vi "Resistomat_2316_2.vi"(0 "Scala resistomat":u16(ring)=5 items=["2 mOhm", "20 mOhm", "200 mOhm", "2 Ohm", "20 Ohm", "200 Ohm", "2 KOhm", "20 KOhm", "200 KOhm"], 1 "instrument ID":i32, 2 "N meas stab":i32=10, 3 "Precisione":dbl=0.005 format="%#_13g", 4 "T after start":u32=11, 5 "Time bef err":dbl=3.0, 7 "error out":errorcluster, 8 "COM-Port (0)":i32=3 min=1 max=32 step=1, 12 "Sing?":bool) -> (20 "seconds since 1Jan1904":timestamp, 21 "Measuring Value (ohm)":dbl, 25 "errore resistomat":bool, 27 "error out 2":errorcluster)   [LabVIEW 2019]
uses:
  Stop lettura res.vi
panel:
  in  "milliseconds to wait":u32=100
  out "Instrument Answers":string
  in  "Numeric 2":i32=5
  out "Numeric":i32
  in  "ms to wait":u32=100
  out "Measuring Value":dbl
  in  "array misure":dbl[](array[numeric])
  out "Scala resistomat 2":u16
  out "t":i32
  out "x .and. y?":bool
  out "x-y":dbl
  out "questionable status register":bool[](array[boolean])
  out "oper status register":bool[](array[boolean])
  out "error":bool
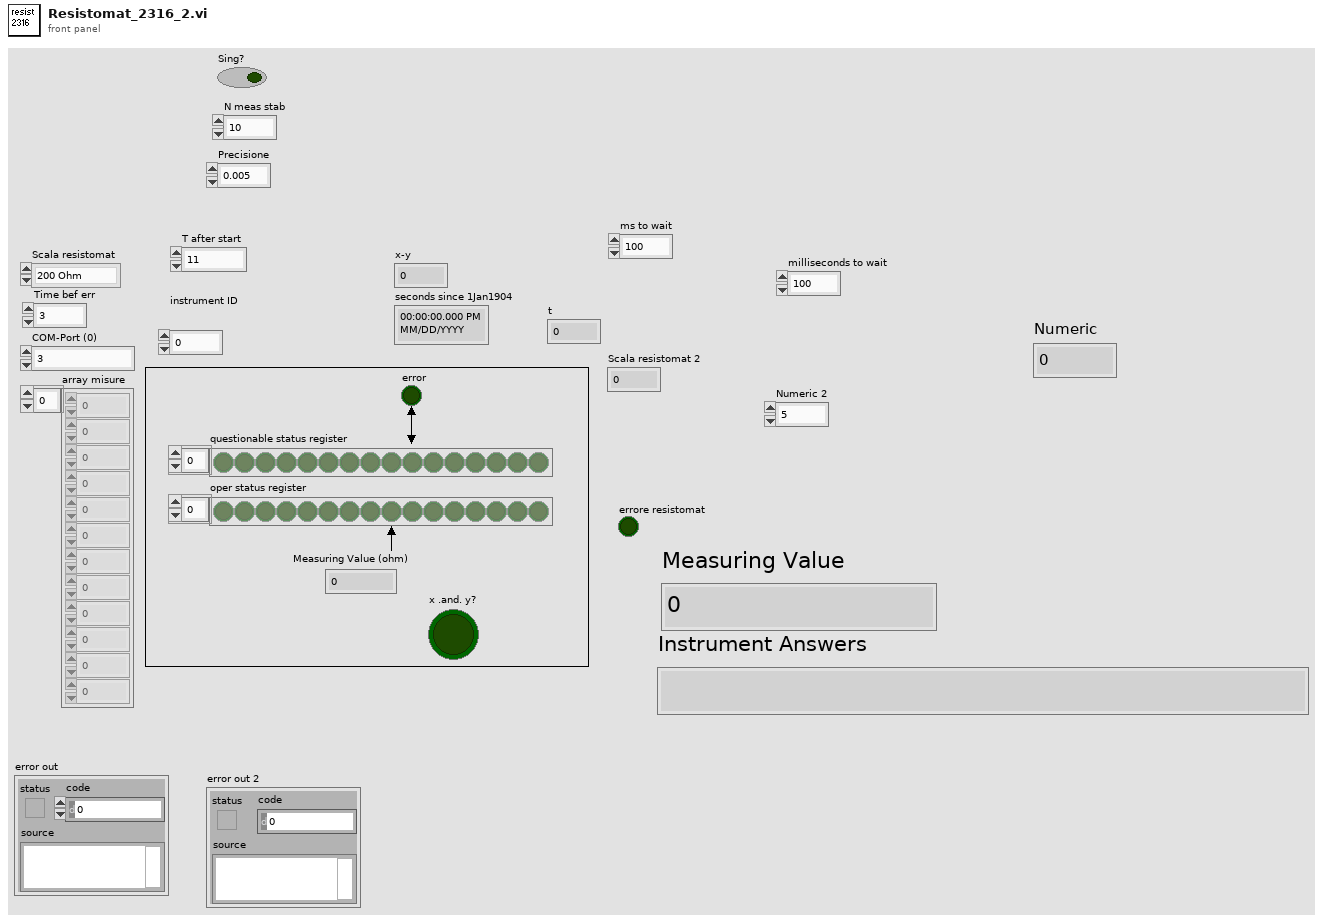
[diagram p1: front panel]
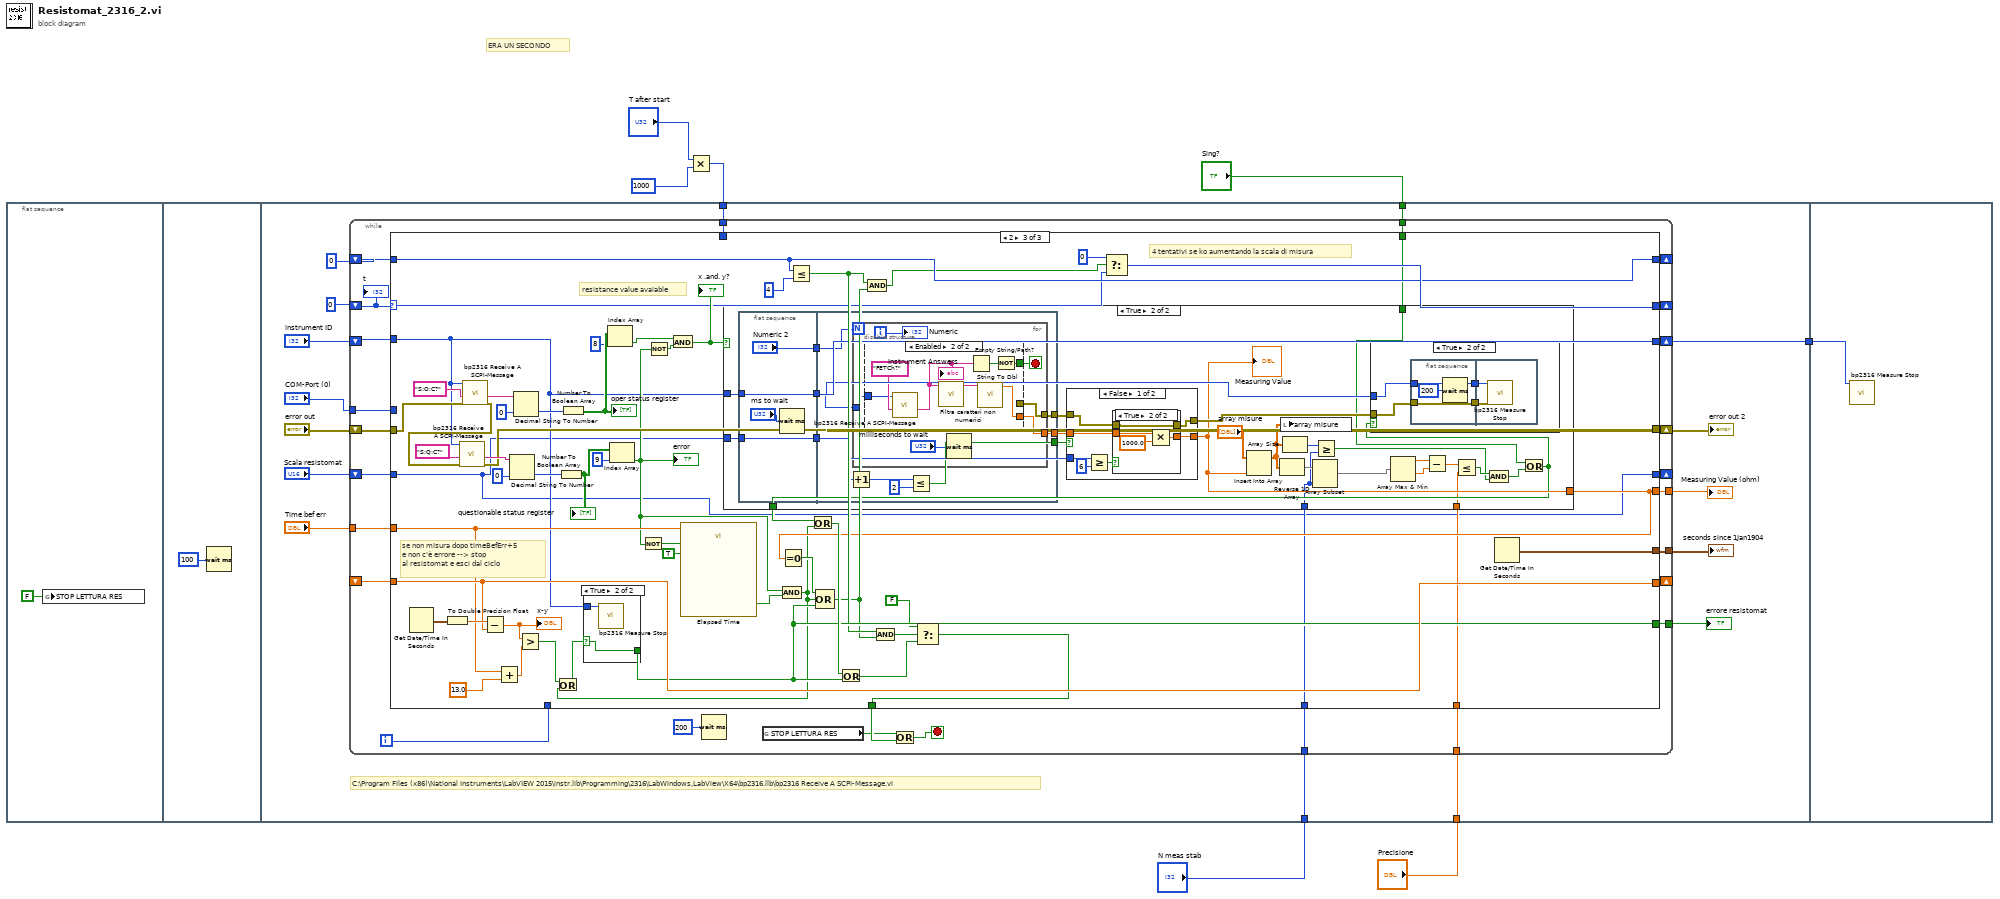
[diagram p0: block diagram]
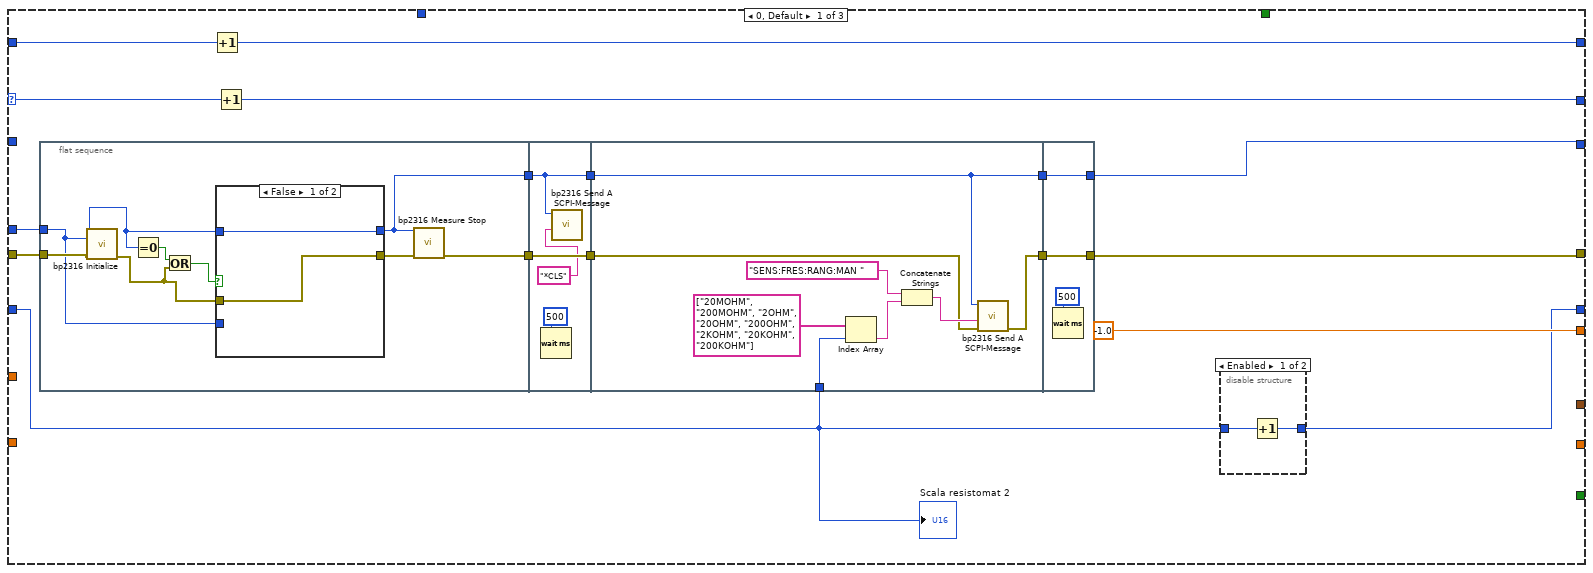
[diagram p2: hidden frame]
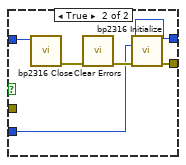
[diagram p4: hidden frame]
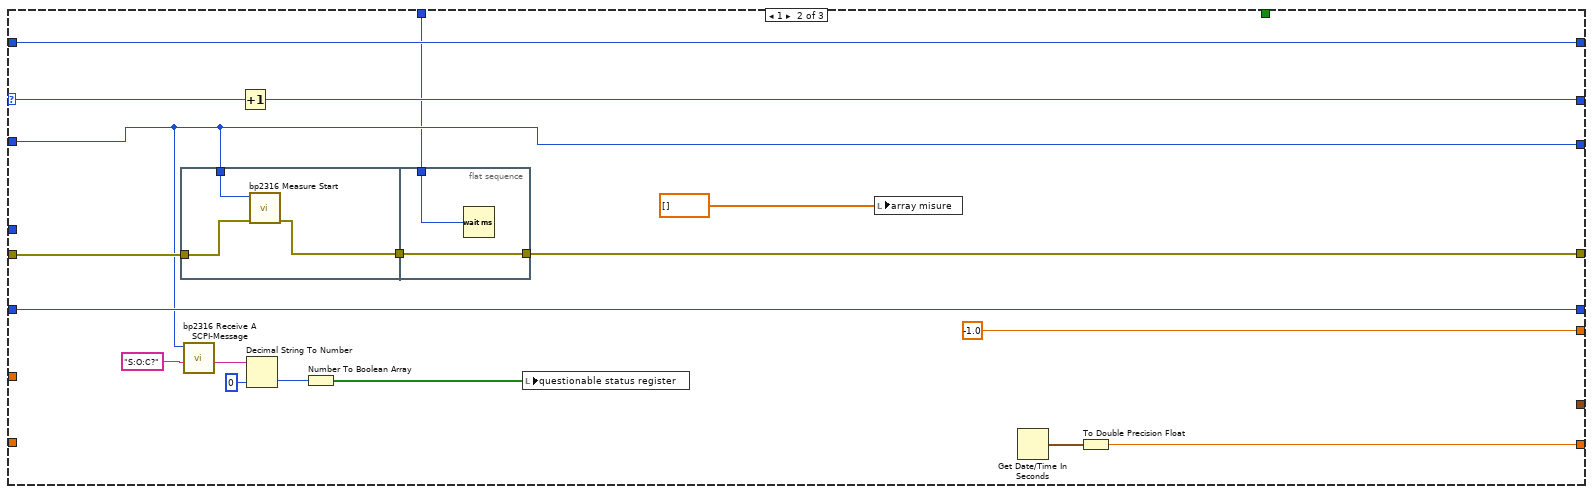
[diagram p5: hidden frame]
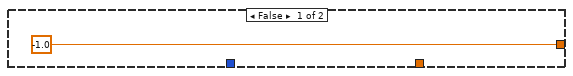
[diagram p7: hidden frame]
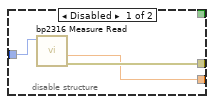
[diagram p9: hidden frame]
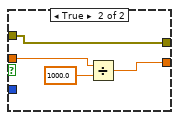
[diagram p11: hidden frame]
diagram:
  # "ERA UN SECONDO"
  n1 = flat-sequence {
    tunnel: [w14] -> w7
    tunnel: "Sing?" -> [w13]
    tunnel: w1 -> [w12]
    tunnel: "N meas stab" -> [w11]
    tunnel: "Precisione" -> [w10]
    tunnel: w7 -> [w264]
    frame #0 {
      n2 = global write "Stop lettura res.vi" "STOP LETTURA RES"(FALSE ("STOP LETTURA RES")) -> ()
    }
    frame #1 {
      n3 = Wait (ms)(milliseconds to wait=u32 100) -> ()  [unwired: 1 out]
    }
    frame #2 {
      # "C:\\Program Files (x86)\\National Instruments\\LabVIEW 2015\\instr.lib\\Programming\\2316\\LabWindows,LabView\\X64\\bp2316.llb\\bp2316 Receive A SCPI-Message.vi"
      n4 = while {
        shift-right: [w48] -> _
        shift-left: 0 -> [w51]
        shift-right: [w50] -> w14
        shift-left: "instrument ID" -> [w49]
        shift-right: [w46] -> w23
        shift-left: "error out" -> [w45]
        tunnel: [w44] -> w21
        shift-right: [w43] -> _
        shift-left: _ -> [w42]
        tunnel: [w41] -> w20
        tunnel: "Time bef err" -> [w39]
        tunnel: [w38] -> w17
        shift-right: [w35] -> _
        shift-left: 0 -> [w36]
        tunnel: "COM-Port (0)" -> [w32]
        shift-right: [w30] -> _
        shift-left: "Scala resistomat" -> [w40]
        tunnel: w13 -> [w29]
        tunnel: w12 -> [w28]
        tunnel: w11 -> [w27]
        tunnel: w10 -> [w26]
        i -> [w37]
        stop <- w33 stop-if-true
        n5 = case shown="2" w51 {
          selector: w51 -> [w68 w121 w135]
          tunnel: [w60 w107 w132] -> w50
          tunnel: w49 -> [_ w107 w132]
          tunnel: [w67 w120 w148] -> w48
          tunnel: [w63 w118 w151] -> w46
          tunnel: w45 -> [w62 w119 w155]
          tunnel: [_ _ w142] -> w34
          tunnel: [-1.0 ("Measuring Value") -1.0 ("Measuring Value") w137] -> w44
          tunnel: [_ w115 w165] -> w43
          tunnel: w42 -> [_ _ w165]
          tunnel: [_ _ w145] -> w41
          tunnel: w40 -> [w52 w113 w128]
          tunnel: w39 -> [_ _ w161]
          tunnel: [_ _ w153] -> w38
          tunnel: w37 -> [_ _ _]
          tunnel: w36 -> [w65 w114 w147]
          tunnel: [w64 w114 w147] -> w35
          tunnel: w32 -> [w61 _ _]
          tunnel: [w53 w113 w128] -> w30
          tunnel: w29 -> [_ _ w131]
          tunnel: w28 -> [_ w104 _]
          tunnel: w27 -> [_ _ w130]
          tunnel: w26 -> [_ _ w129]
          frame 0, Default {
            n6 = flat-sequence {
              tunnel: w62 -> [w79]
              tunnel: w61 -> [w73]
              tunnel: [w80] -> w59
              tunnel: [w78] -> w58
              tunnel: w59 -> [w92]
              tunnel: w58 -> [w90]
              tunnel: [w92] -> w55
              tunnel: [w90] -> w54
              tunnel: w52 -> [w94]
              tunnel: [w95] -> w57
              tunnel: [w97] -> w56
              tunnel: w55 -> [w93]
              tunnel: w54 -> [w97]
              tunnel: [w102] -> w60
              tunnel: [w103] -> w63
              tunnel: w57 -> [w103]
              tunnel: w56 -> [w102]
              frame #0 {
                n7 = call <instrlib>:"bp2316 Initialize.vi"("COM-Port (0)"=w73, "error in (no error)"=w79) -> ("Instrument ID"=w72:i32, "error out"=w74:errorcluster)  [unwired: 11 in, 1 out]
                n8 = Equal To 0?(x=w72) -> (x = 0?=w76:bool)
                n9 = Or(x=w76, y=w74) -> (x .or. y?=w75:bool)
                n10 = case shown="False" w75 {
                  tunnel: w72 -> [w82 w87]
                  tunnel: w73 -> [_ w84]
                  tunnel: [w81 w88] -> w77
                  tunnel: [w82 w83] -> w78
                  tunnel: w74 -> [w81 _]
                  frame False {
                  }
                  frame True {
                    n11 = call <instrlib>:"bp2316 Close.vi"("Instrument ID (1)"=w87) -> ("error out"=w86:errorcluster)  [unwired: 9 in, 1 out]
                    n12 = call <vilib>:"Clear Errors.vi"("error in (no error)"=w86) -> ("error out"=w85:errorcluster)  [unwired: 5 in, 1 out]
                    n13 = call <instrlib>:"bp2316 Initialize.vi"("COM-Port (0)"=w84, "error in (no error)"=w85) -> ("Instrument ID"=w83:i32, "error out"=w88:errorcluster)  [unwired: 11 in, 1 out]
                  }
                }
                n14 = call <instrlib>:"bp2316 Measure Stop.vi"("error in (no error)"=w77, "Instrument ID (1)"=w78) -> ("error out"=w80:errorcluster)  [unwired: 8 in, 1 out]
              }
              frame #1 {
                n15 = Wait (ms)(milliseconds to wait=u32 500) -> ()  [unwired: 1 out]
                n16 = call <instrlib>:"bp2316 Send A SCPI-Message.vi"("Send-SCPI-Message"="*CLS" ("sendSCPIMessage"), "Instrument ID (1)"=w90) -> ()  [unwired: 8 in, 2 out]
              }
              frame #2 {
                n17 = Index Array(array=string[] ["20MOHM", "200MOHM", "2OHM", "20OHM", "200OHM", "2KOHM", "20KOHM", "200KOHM"], index=w94) -> (element=w98:string)
                n18 = Concatenate Strings("SENS:FRES:RANG:MAN " ("sendSCPIMessage"), w98) -> (w96:string)
                n19 = call <instrlib>:"bp2316 Send A SCPI-Message.vi"("error in (no error)"=w93, "Send-SCPI-Message"=w96, "Instrument ID (1)"=w97) -> ("error out"=w95:errorcluster)  [unwired: 7 in, 1 out]
              }
              frame #3 {
                n20 = Wait (ms)(milliseconds to wait=u32 500) -> ()  [unwired: 1 out]
              }
            }
            n21 = Increment(x=w65) -> (x+1=w64:i32)
            n22 = Increment(x=w68) -> (x+1=w67:i32)
            n23 = disable-structure shown="Enabled" {
              disable-tunnel: [w70 w71] -> w53
              disable-tunnel: w52 -> [w69 w71]
              frame Enabled {
                n24 = Increment(x=w69) -> (x+1=w70:u16)
              }
              frame Disabled {
              }
            }
            "Scala resistomat 2" <- w52
          }
          frame 1 {
            n25 = flat-sequence {
              tunnel: w107 -> [w124]
              tunnel: w119 -> [w123]
              tunnel: [w122] -> w112
              tunnel: [w126] -> w118
              tunnel: w112 -> [w126]
              tunnel: w104 -> [w125]
              frame #0 {
                n26 = call <instrlib>:"bp2316 Measure Start.vi"("error in (no error)"=w123, "Instrument ID (1)"=w124) -> ("error out"=w122:errorcluster)  [unwired: 8 in, 1 out]
              }
              frame #1 {
                n27 = Wait (ms)(milliseconds to wait=w125) -> ()  [unwired: 1 out]
              }
            }
            n28 = call <instrlib>:"bp2316 Receive A SCPI-Message.vi"("Send-SCPI-Message"="S:O:C?" ("sendSCPIMessage"), "Instrument ID (1)"=w107) -> ("Instrument Answers"=w109:string)  [unwired: 7 in, 2 out]
            n29 = Increment(x=w121) -> (x+1=w120:i32)
            n30 = Decimal String To Number(string=w109, default (0L)=i16 0 ("default (0 I32)")) -> (number=w111:i16)  [unwired: 1 in, 1 out]
            n31 = Number To Boolean Array(number=w111) -> (Boolean array=w106:bool[])
            n32 = local write "questionable status register"(w106) -> ()
            n33 = local write "array misure"(dbl[] [] ("array misure")) -> ()
            n34 = Get Date/Time In Seconds() -> (seconds since 1Jan1904=w116:timestamp)
            n35 = To Double Precision Float(number=w116) -> (double precision float=w115:dbl)
          }
          frame 2 {
            # "4 tentativi se ko aumentando la scala di misura"
            # "se non misura dopo timeBefErr+5\ne non c'è errore --> stop\nal resistomat e esci dal ciclo"
            # "resistance value avaiable"
            n36 = Get Date/Time In Seconds() -> (seconds since 1Jan1904=w167:timestamp)
            n37 = To Double Precision Float(number=w167) -> (double precision float=w166:dbl)
            n38 = call <instrlib>:"bp2316 Receive A SCPI-Message.vi"("error in (no error)"=w155, "Send-SCPI-Message"="S:O:C?" ("sendSCPIMessage"), "Instrument ID (1)"=w132) -> ("error out"=w152:errorcluster, "Instrument Answers"=w158:string)  [unwired: 6 in, 1 out]
            n39 = call <instrlib>:"bp2316 Receive A SCPI-Message.vi"("error in (no error)"=w152, "Send-SCPI-Message"="S:Q:C?" ("sendSCPIMessage"), "Instrument ID (1)"=w132) -> ("error out"=w151:errorcluster, "Instrument Answers"=w154:string)  [unwired: 6 in, 1 out]
            n40 = Subtract(x=w166, y=w165) -> (x-y=w164:dbl)
            "x-y" <- w164
            n41 = Add(x=w161, y=13.0) -> (x+y=w162:dbl)
            n42 = Decimal String To Number(string=w154, default (0L)=i16 0 ("default (0 I32)")) -> (number=w175:i16)  [unwired: 1 in, 1 out]
            n43 = Decimal String To Number(string=w158, default (0L)=i16 0 ("default (0 I32)")) -> (number=w178:i16)  [unwired: 1 in, 1 out]
            n44 = Greater?(x=w164, y=w162) -> (0:w134:bool)
            n45 = Number To Boolean Array(number=w175) -> (Boolean array=w173:bool[])
            "questionable status register" <- w173
            n46 = Number To Boolean Array(number=w178) -> (Boolean array=w181:bool[])
            "oper status register" <- w181
            n47 = Index Array(array=w181, index=8) -> (element=w174:bool)
            n48 = Index Array(array=w173, index=9) -> (element=w146:bool)
            "error" <- w146
            n49 = Not(x=w146) -> (.not. x?=w168:bool)
            n50 = Not(x=w146) -> (.not. x?=w172:bool)
            n51 = And(x=w174, y=w172) -> (x .and. y?=w159:bool)
            "x .and. y?" <- w159
            n52 = call "Elapsed Time"("Time Target (s)"=w161, "Reset"=w168, "Auto Reset"=TRUE) -> ("Time has Elapsed"=w170:bool)  [unwired: 9 in, 7 out]
            n53 = case shown="True" w159 {
              tunnel: w132 -> [_ w206]
              tunnel: [_ w189] -> w171
              tunnel: [-1.0 ("Measuring Value") w200] -> w137
              tunnel: w128 -> [_ w207]
              tunnel: w131 -> [_ w186]
              tunnel: w130 -> [_ w188]
              tunnel: w129 -> [_ w187]
              frame False {
              }
              frame True {
                n54 = flat-sequence {
                  tunnel: w206 -> [w221]
                  tunnel: w207 -> [w222]
                  tunnel: [w222] -> w203
                  tunnel: [w221] -> w202
                  tunnel: ["Numeric 2"] -> w185
                  tunnel: [w229] -> w209
                  tunnel: [w228] -> w208
                  tunnel: [w226] -> w205
                  tunnel: w203 -> [w225]
                  tunnel: w202 -> [w227]
                  tunnel: w185 -> [w223]
                  frame #0 {
                    n55 = Wait (ms)(milliseconds to wait="ms to wait") -> ()  [unwired: 1 out]
                  }
                  frame #1 {
                    n56 = Increment(x=w225) -> (x+1=w224:u16)
                    n57 = for {
                      N: w223 -> [_]
                      tunnel: [w234] -> w228
                      tunnel: w227 -> [w236]
                      tunnel: [w235] -> w226
                      i -> [w232]
                      stop <- w231 stop-if-true
                      n58 = disable-structure shown="Enabled" {
                        disable-tunnel: w236 -> [w239 w245]
                        disable-tunnel: [w238 _] -> w235
                        disable-tunnel: [w237 w244] -> w234
                        disable-tunnel: [_ w242] -> w231
                        frame Disabled {
                          n59 = call <instrlib>:"bp2316 Measure Read.vi"("Instrument ID (1)"=w239) -> ("error out"=w238:errorcluster, "Measuring Value"=w237:dbl)  [unwired: 7 in, 2 out]
                        }
                        frame Enabled {
                          n60 = call <instrlib>:"bp2316 Receive A SCPI-Message.vi"("Send-SCPI-Message"="FETCh?" ("sendSCPIMessage"), "Instrument ID (1)"=w245) -> ("Instrument Answers"=w241:string)  [unwired: 7 in, 2 out]
                          "Instrument Answers" <- w241
                          n61 = call "Filtra caratteri non numerici.vi"("string in"=w241) -> ("string"=w240:string)  [unwired: 10 in]
                          n62 = Empty String/Path?(string/path=w241) -> (empty?=w243:bool)
                          n63 = call "String To Dbl.vi"("String"=w240) -> ("Numeric"=w244:dbl)  [unwired: 10 in]
                          n64 = Not(x=w243) -> (.not. x?=w242:bool)
                        }
                      }
                      n65 = Wait (ms)(milliseconds to wait="milliseconds to wait") -> ()  [unwired: 1 out]
                      "Numeric" <- w232
                    }
                    n66 = Less Or Equal?(x=w224, y=u16 2) -> (x <= y?=w229:bool)
                  }
                }
                n67 = case shown="False" w209 {
                  tunnel: w208 -> [w250 w263]
                  tunnel: [w249 w261] -> w200
                  tunnel: w207 -> [w253 _]
                  tunnel: w205 -> [w248 w260]
                  tunnel: [w247 w260] -> w204
                  frame False {
                    n68 = Greater Or Equal?(x=w253, y=u16 6) -> (x >= y?=w251:bool)
                    n69 = case shown="True" w251 {
                      tunnel: w250 -> [w255 w259]
                      tunnel: [w255 w257] -> w249
                      tunnel: w248 -> [w254 w256]
                      tunnel: [w254 w256] -> w247
                      frame False {
                      }
                      frame True {
                        n70 = Multiply(x=w259, y=1000.0) -> (x*y=w257:dbl)
                      }
                    }
                  }
                  frame True {
                    n71 = Divide(x=w263, y=1000.0) -> (x/y=w261:dbl)
                  }
                }
                "Measuring Value" <- w200
                n72 = Insert Into Array(array="array misure", new element=w200) -> (w194:dbl[])  [unwired: 1 in]
                n73 = Reverse 1D Array(array=w194) -> (reversed array=w199:dbl[])
                n74 = local write "array misure"(w194) -> ()
                n75 = Array Size(array=w194) -> (size(s)=w193:i32)
                n76 = Array Subset(array=w199, length=w188) -> (w198:dbl[])  [unwired: 1 in]
                n77 = Greater Or Equal?(x=w193, y=w188) -> (x >= y?=w191:bool)
                n78 = Array Max & Min(array=w198) -> (max value=w197:dbl, min value=w196:dbl)  [unwired: 2 out]
                n79 = Subtract(x=w197, y=w196) -> (x-y=w195:dbl)
                n80 = Less Or Equal?(x=w195, y=w187) -> (x <= y?=w192:bool)
                n81 = And(x=w192, y=w191) -> (x .and. y?=w190:bool)
                n82 = Or(x=w186, y=w190) -> (x .or. y?=w189:bool)
                n83 = case shown="True" w189 {
                  tunnel: w206 -> [_ w213]
                  tunnel: w204 -> [_ w212]
                  frame False {
                  }
                  frame True {
                    n84 = flat-sequence {
                      tunnel: w212 -> [w215]
                      tunnel: w213 -> [w216]
                      tunnel: [w216] -> w211
                      tunnel: [w215] -> w210
                      tunnel: w211 -> [w218]
                      tunnel: w210 -> [w217]
                      frame #0 {
                        n85 = Wait (ms)(milliseconds to wait=u32 200) -> ()  [unwired: 1 out]
                      }
                      frame #1 {
                        n86 = call <instrlib>:"bp2316 Measure Stop.vi"("error in (no error)"=w217, "Instrument ID (1)"=w218) -> ()  [unwired: 8 in, 2 out]
                      }
                    }
                  }
                }
              }
            }
            n87 = And(x=w146, y=w170) -> (x .and. y?=w127:bool)
            n88 = Or(x=w134, y=w127) -> (x .or. y?=w133:bool)
            n89 = case shown="True" w133 {
              selector: w133 -> [_ w182]
              tunnel: w132 -> [_ w183]
              tunnel: [_ w182] -> w145
              frame False {
              }
              frame True {
                n90 = call <instrlib>:"bp2316 Measure Stop.vi"("Instrument ID (1)"=w183) -> ()  [unwired: 9 in, 2 out]
              }
            }
            n91 = Equal To 0?(x=w137) -> (x = 0?=w136:bool)
            n92 = Less Or Equal?(x=w147, y=4) -> (x <= y?=w140:bool)
            n93 = Or(x=w171, y=w127) -> (x .or. y?=w163:bool)
            n94 = Compound Arithmetic op=OR(w136, w127, w145) -> (w139:bool)
            n95 = Or(x=w163, y=w145) -> (x .or. y?=w143:bool)
            n96 = And(x=w140, y=w139) -> (x .and. y?=w138:bool)
            n97 = And(x=w140, y=w139) -> (x .and. y?=w144:bool)
            n98 = Select(t=FALSE, s=w144, f=w143) -> (s? t:f=w142:bool)
            n99 = Select(t=0, s=w138, f=w135) -> (s? t:f=w148:i32)
            n100 = Get Date/Time In Seconds() -> (seconds since 1Jan1904=w153:timestamp)
          }
        }
        n101 = Wait (ms)(milliseconds to wait=u32 200) -> ()  [unwired: 1 out]
        n102 = global read "Stop lettura res.vi" "STOP LETTURA RES"() -> (w31:bool)
        n103 = Or(x=w31, y=w34) -> (x .or. y?=w33:bool)
        "t" <- w51
      }
      "error out 2" <- w23
      "Measuring Value (ohm)" <- w21
      "errore resistomat" <- w20
      "seconds since 1Jan1904" <- w17
    }
    frame #3 {
      n104 = call <instrlib>:"bp2316 Measure Stop.vi"("Instrument ID (1)"=w264) -> ()  [unwired: 9 in, 2 out]
    }
  }
  n105 = Multiply(x="T after start", y=u32 1000) -> (x*y=w1:u32)
